vi "InterpolateScanPoints.vi"(8 "error in (no error)":errorcluster, 9 "Parameters":T1={"number of planes"=4, "z step"=1.9999999999999998e-05, "pixel dwell time"=1.0000000000000001e-11, "z frequency"=10.0, "number of pixels"=100, "smooth points"=10, "smooth line"=10, "Sine\nSawtooth"=FALSE, "PointSorting"=0, "Sort Points"=FALSE, "X-pixels"=256.0, "Y-lines"=256.0, "pixelstoµm"=256.0, "zoom"=1.0, "Time offset"=1.0000000000000001e-11} {"zoom" min=0.5 step=0.1; "Y-lines" min=1 step=1; "X-pixels" min=1 step=1; "PointSorting" items=["No Difference", "Every Second Point", "Down / Up"]; "smooth line" min=1; "smooth points" min=1; "number of pixels" min=1; "z frequency" format="%_4g"; "number of planes" min=1}, 10 "DutyCluster":T2 {"Iteration" items=["first iteration", "second iteration"]}, 11 "x pixels, y pixels, z, time":dbl[][](array[numeric])) -> (0 "error out":errorcluster, 1 "Parameters":T1={"number of planes"=4, "z step"=1.9999999999999998e-05, "pixel dwell time"=1.0000000000000001e-11, "z frequency"=10.0, "number of pixels"=100, "smooth points"=10, "smooth line"=10, "Sine\nSawtooth"=FALSE, "PointSorting"=0, "Sort Points"=FALSE, "X-pixels"=256.0, "Y-lines"=256.0, "pixelstoµm"=256.0, "zoom"=1.0, "Time offset"=1.0000000000000001e-11} {"zoom" min=0.5 step=0.1; "Y-lines" min=1 step=1; "X-pixels" min=1 step=1; "PointSorting" items=["No Difference", "Every Second Point", "Down / Up"]; "smooth line" min=1; "smooth points" min=1; "number of pixels" min=1; "z frequency" format="%_4g"; "number of planes" min=1}, 2 "DutyCluster":T2 {"Iteration" items=["first iteration", "second iteration"]}, 3 "x pixels, y pixels, z, time":dbl[][](array[numeric]))   [LabVIEW 2010]
uses:
  TypeDefs/DutyCluster.ctl
  TypeDefs/ParameterCluster.ctl
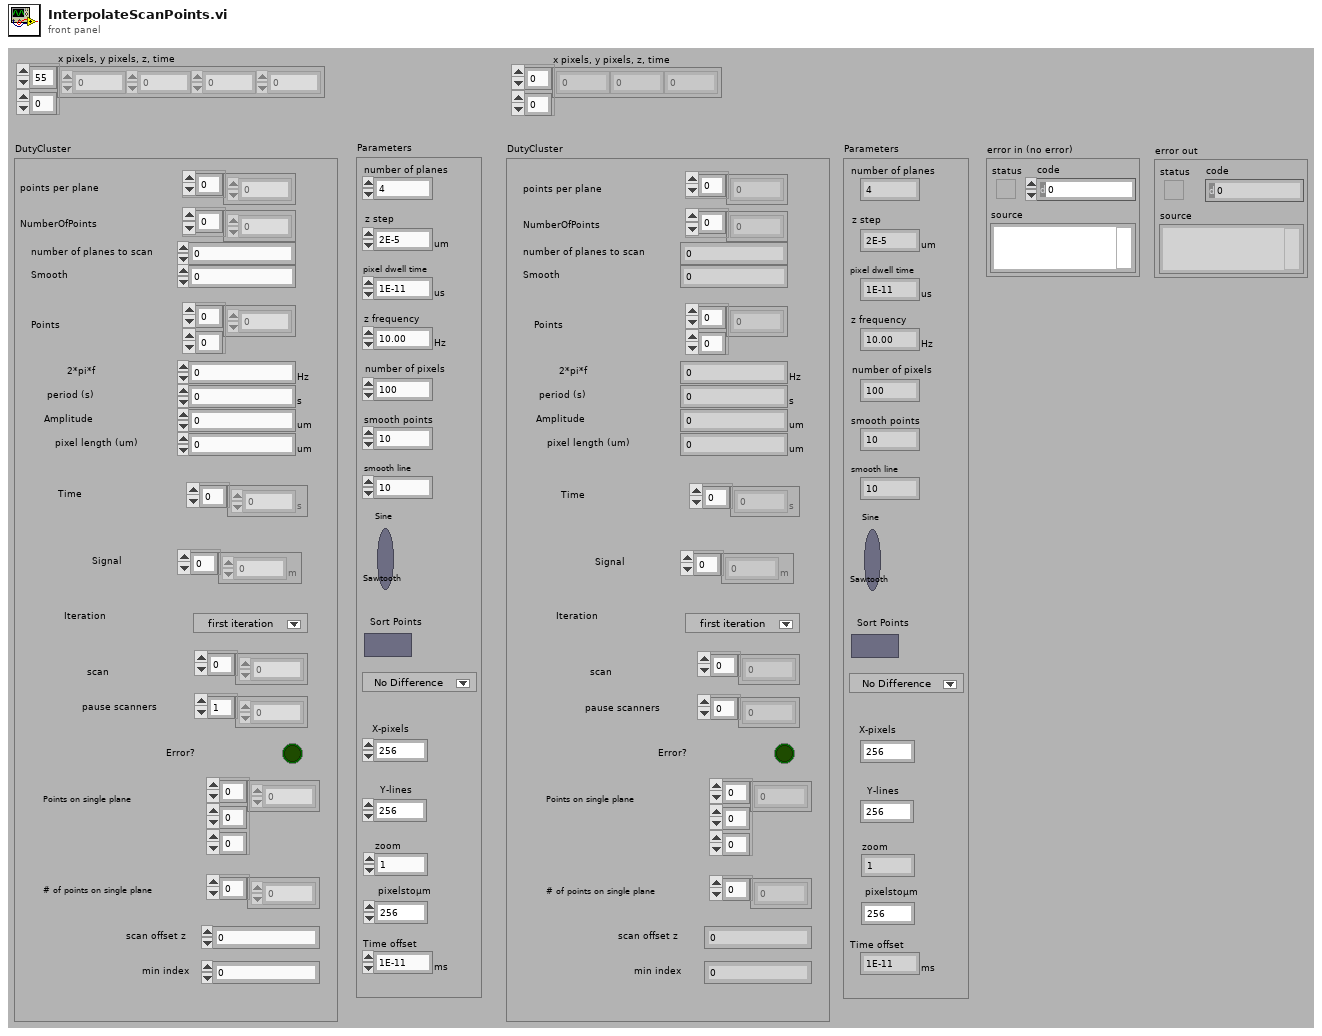
[diagram p1: front panel]
types:
  T1 = typedef "ParameterCluster.ctl" = cluster{"number of planes":i32, "z step":dbl[unit], "pixel dwell time":dbl[unit], "z frequency":dbl[unit], "number of pixels":i32, "smooth points":i32, "smooth line":i32, "Sine\nSawtooth":bool, "PointSorting":u16, "Sort Points":bool, "X-pixels":sgl, "Y-lines":sgl, "pixelstoµm":dbl, "zoom":dbl, "Time offset":dbl[unit]}
  T2 = typedef "DutyCluster.ctl" = cluster{"points per plane":i32[], "NumberOfPoints":i32[], "number of planes to scan":i32, "Smooth":i32, "Points":dbl[][], "2*pi*f":dbl[unit], "period (s)":dbl[unit], "Amplitude":dbl[unit], "pixel length (um)":dbl[unit], "Time":dbl[unit][], "Signal":dbl[unit][], "Iteration":u16, "scan":i32[], "pause scanners":i32[], "Error?":bool, "Points on single plane":dbl[][][], "# of points on single plane":i32[], "scan offset z":i32, "min index":i32}
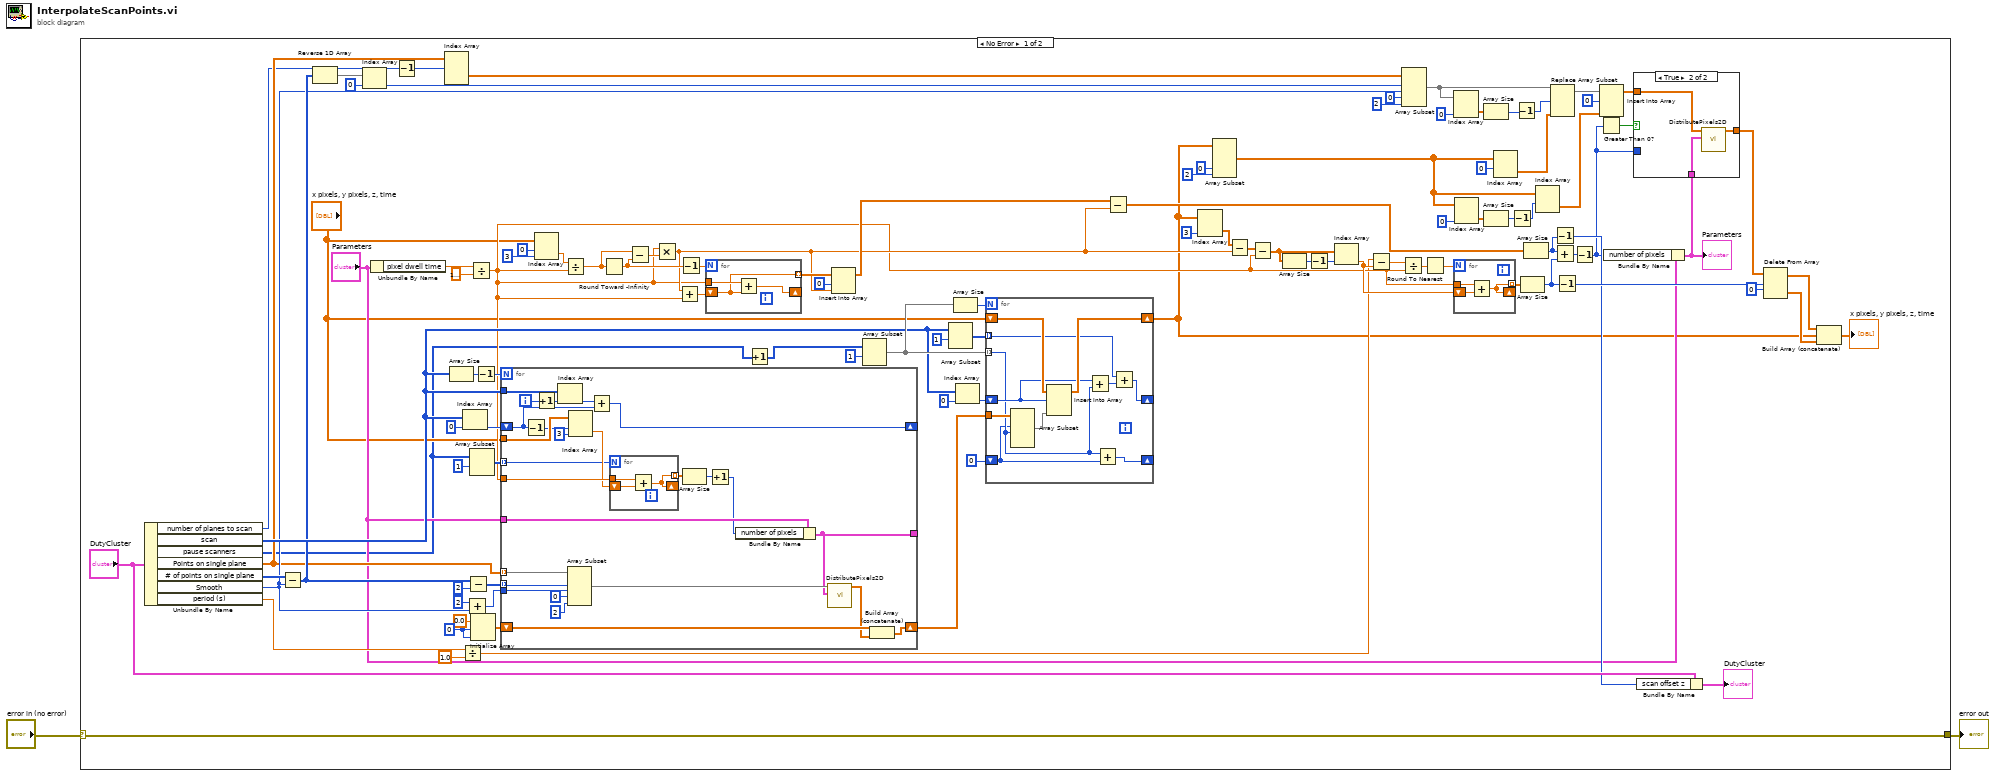
[diagram p0: block diagram]
diagram:
  n1 = case shown="No Error" "error in (no error)" {
    selector: "error in (no error)" -> [w10 w157]
    tunnel: [w10 w157] -> w1
    frame No Error {
      w54 = 0 ("dimension size")
      n2 = Unbundle By Name("DutyCluster") -> ("number of planes to scan"=w18:i32, "scan"=w55:i32[], "pause scanners"=w5:i32[], "Points on single plane"=w19:dbl[][][], "# of points on single plane"=w23:i32[], "Smooth"=w21:i32, "period (s)"=w27:dbl[unit])
      n3 = Subtract(x=w23, y=w21) -> (x-y=w22:i32[])
      n4 = Reverse 1D Array(array=w22) -> (reversed array=w25:i32[])
      n5 = Index Array(array=w25, index=0) -> (element=w20:i32)
      n6 = Unbundle By Name("Parameters") -> ("pixel dwell time"=w30:dbl[unit])
      n7 = Decrement(x=w18) -> (x-1=w17:i32)
      n8 = Index Array(array=w19, index (dim 0)=w17) -> (element=w16:dbl[][])  [unwired: 2 in]
      n9 = Array Size(array=w55) -> (size(s)=w69:i32)
      n10 = Divide(x=w27, y=dbl[unit] 1.0) -> (x/y=w26:dbl)
      n11 = Index Array(array=w55, index=0) -> (element=w96:i32)
      n12 = Add(x=2, y=w21) -> (x+y=w67:i32)
      n13 = Subtract(x=w22, y=2) -> (x-y=w71:i32[])
      n14 = Divide(x=w30, y=dbl[unit] 1e-06) -> (x/y=w29:dbl)
      n15 = Array Subset(array=w5, index=1) -> (w99:i32[])  [unwired: 1 in]
      n16 = Initialize Array(0.0 ("element"), w54, w54) -> (w73:dbl[][])
      n17 = Decrement(x=w69) -> (x-1=w68:i32)
      n18 = for {
        N: w68 -> [_]
        tunnel: w55 -> [w149]
        tunnel: "x pixels, y pixels, z, time" -> [w138]
        tunnel: w99 -> [w131] mode=indexing
        tunnel: w29 -> [w133]
        shift-right: [w142] -> _
        shift-left: w96 -> [w135]
        shift-right: [w136] -> w6
        shift-left: w73 -> [w141]
        tunnel: w19 -> [w140] mode=indexing
        tunnel: w71 -> [w137] mode=indexing
        tunnel: w67 -> [w139]
        tunnel: "Parameters" -> [w128]
        tunnel: [w125] -> _
        i -> [w147]
        n19 = Decrement(x=w135) -> (x-1=w134:i32)
        n20 = Increment(x=w147) -> (x+1=w146:i32)
        n21 = Index Array(array=w149, index=w146) -> (element=w148:i32)
        n22 = Array Subset(array=w140, index (row)=w137, length (row)=w139, index (col)=0 ("index"), length (col)=2 ("length")) -> (w129:dbl[][])
        n23 = Index Array(array=w138, index (row)=w134, index (col)=3 ("index")) -> (element=w132:dbl)
        n24 = Add(x=w148, y=w135) -> (x+y=w142:i32)
        n25 = for {
          N: w131 -> [_]
          shift-right: [w151] -> _
          shift-left: w132 -> [w152]
          tunnel: w133 -> [w153]
          tunnel: [w151] -> w143 mode=indexing
          n26 = Add(x=w153, y=w152) -> (x+y=w151:dbl)
        }
        n27 = Array Size(array=w143) -> (size(s)=w130:i32)
        n28 = Increment(x=w130) -> (x+1=w127:i32)
        n29 = Bundle By Name(cluster=w128, "number of pixels"=w127) -> (w125:T1)
        n30 = call "DistributePixels2D.vi"("Parameters"=w125, "XY coordinates"=w129) -> ("XY coordinates interpolated"=w126:dbl[][])  [unwired: 8 in, 1 out]
        n31 = Build Array (concatenate)(w141, w126) -> (w136:dbl[][])
      }
      n32 = Index Array(array="x pixels, y pixels, z, time", index (row)=0 ("disabled index (row)"), index (col)=3 ("disabled index (col)")) -> (element=w105:dbl)
      n33 = Divide(x=w105, y=w29) -> (x/y=w106:dbl)
      n34 = Round Toward -Infinity(1:w106) -> (0:w101:dbl)
      n35 = Subtract(x=w106, y=w101) -> (x-y=w103:dbl)
      n36 = Multiply(x=w29, y=w103) -> (x*y=w58:dbl)
      n37 = Add(x=w58, y=w29) -> (x+y=w102:dbl)
      n38 = Decrement(x=w101) -> (x-1=w100:dbl)
      n39 = for {
        N: w100 -> [_]
        shift-right: [w155] -> _
        shift-left: w102 -> [w154]
        tunnel: w29 -> [w156]
        tunnel: [w154] -> w86 mode=indexing
        n40 = Add(x=w156, y=w154) -> (x+y=w155:dbl)
      }
      n41 = Increment(x=w5) -> (x+1=w4:i32[])
      n42 = Insert Into Array(array=w86, index=0, new element=w58) -> (w74:dbl[])
      n43 = Array Subset(array=w4, index=1) -> (w90:i32[])  [unwired: 1 in]
      n44 = Array Subset(array=w55, index=1) -> (w88:i32[])  [unwired: 1 in]
      n45 = Array Size(array=w90) -> (size(s)=w89:i32)
      n46 = Index Array(array=w55, index=0) -> (element=w93:i32)
      n47 = for {
        N: w89 -> [_]
        tunnel: w88 -> [w120] mode=indexing
        tunnel: w90 -> [w116] mode=indexing
        shift-right: [w118] -> _
        shift-left: w93 -> [w121]
        tunnel: w6 -> [w124]
        shift-right: [w114] -> _
        shift-left: 0 ("index") -> [w115]
        shift-right: [w122] -> w8
        shift-left: "x pixels, y pixels, z, time" -> [w123]
        n48 = Array Subset(array=w124, index (row)=w115, length (row)=w116) -> (w117:dbl[][])  [unwired: 2 in]
        n49 = Insert Into Array(array=w123, index (row)=w121, new element=w117) -> (w122:dbl[][])  [unwired: 1 in]
        n50 = Add(x=w121, y=w116) -> (x+y=w119:i32)
        n51 = Add(x=w116, y=w115) -> (x+y=w114:i32)
        n52 = Add(x=w120, y=w119) -> (x+y=w118:i32)
      }
      n53 = Subtract(x=w74, y=w58) -> (x-y=w75:dbl[])
      n54 = Index Array(array=w8, index (col)=3 ("index")) -> (element=w84:dbl[])  [unwired: 1 in]
      n55 = Array Subset(array=w8, index (col)=0 ("index"), length (col)=2 ("length")) -> (w32:dbl[][])  [unwired: 2 in]
      n56 = Subtract(x=w84, y=w58) -> (x-y=w61:dbl[])
      n57 = Subtract(x=w61, y=w29) -> (x-y=w60:dbl[])
      n58 = Array Size(array=w60) -> (size(s)=w83:i32)
      n59 = Decrement(x=w83) -> (x-1=w82:i32)
      n60 = Index Array(array=w60, index=w82) -> (element=w79:dbl)
      n61 = Subtract(x=w26, y=w79) -> (x-y=w80:dbl)
      n62 = Divide(x=w80, y=w29) -> (x/y=w81:dbl)
      n63 = Array Subset(array=w16, index (row)=w20, length (row)=w21, index (col)=0 ("index"), length (col)=2 ("length")) -> (w41:dbl[][])
      n64 = Round To Nearest(number=w81) -> (nearest integer value=w59:dbl)
      n65 = Index Array(array=w41, index (col)=0 ("index (row)")) -> (element=w45:dbl[])  [unwired: 1 in]
      n66 = for {
        N: w59 -> [_]
        shift-right: [w111] -> _
        shift-left: w79 -> [w112]
        tunnel: w29 -> [w113]
        tunnel: [w111] -> w76 mode=indexing
        n67 = Add(x=w113, y=w112) -> (x+y=w111:dbl)
      }
      n68 = Index Array(array=w32, index (col)=0 ("index (row)")) -> (element=w65:dbl[])  [unwired: 1 in]
      n69 = Array Size(array=w45) -> (size(s)=w39:i32)
      n70 = Array Size(array=w65) -> (size(s)=w66:i32)
      n71 = Index Array(array=w32, index (row)=0) -> (element=w35:dbl[])  [unwired: 1 in]
      n72 = Decrement(x=w66) -> (x-1=w63:i32)
      n73 = Decrement(x=w39) -> (x-1=w38:i32)
      n74 = Array Size(array=w76) -> (size(s)=w57:i32)
      n75 = Array Size(array=w75) -> (size(s)=w56:i32)
      n76 = Index Array(array=w32, index (row)=w63) -> (element=w33:dbl[])  [unwired: 1 in]
      n77 = Replace Array Subset(array=w41, new element=w35, index (row)=w38) -> (w40:dbl[][])  [unwired: 1 in]
      n78 = Decrement(x=w56) -> (x-1=w14:i32)
      n79 = Add(x=w56, y=w57) -> (x+y=w62:i32)
      n80 = Decrement(x=w57) -> (x-1=w31:i32)
      n81 = Decrement(x=w62) -> (x-1=w13:i32)
      n82 = Insert Into Array(array=w40, index (row)=0, new element=w33) -> (w42:dbl[][])  [unwired: 1 in]
      n83 = Greater Than 0?(x=w13) -> (x > 0?=w34:bool)
      n84 = Bundle By Name(cluster="Parameters", "number of pixels"=w13) -> (w12:T1)
      "Parameters" <- w12
      n85 = case shown="True" w34 {
        tunnel: [w107 w109] -> w47
        tunnel: w42 -> [w107 w110]
        tunnel: w13 -> [_ _]
        tunnel: w12 -> [_ w108]
        frame False {
        }
        frame True {
          n86 = call "DistributePixels2D.vi"("Parameters"=w108, "XY coordinates"=w110) -> ("XY coordinates interpolated"=w109:dbl[][])  [unwired: 8 in, 1 out]
        }
      }
      n87 = Bundle By Name(cluster="DutyCluster", "scan offset z"=w14) -> (→"DutyCluster":T2)
      n88 = Delete From Array(array=w47, length=w31, index (row)=0) -> (deleted portion=w36:dbl[][], array with subset deleted=w37:dbl[][])  [unwired: 1 in]
      n89 = Build Array (concatenate)(w37, w8, w36) -> (→"x pixels, y pixels, z, time":dbl[][])
    }
    frame Error {
    }
  }
  "error out" <- w1
